vi "FipsAdjacent.vi"() -> (11 "Fips":i32[](array[numeric]))   [LabVIEW 2017] (continued)
County, MD\"\t24043\t\"Washington County, MD\"\t24043\n\"Washington County, MD\"\t24043\t\"Franklin County, PA\"\t42055\n\"Washington County, MD\"\t24043\t\"Fulton County, PA\"\t42057\n\"Washington County, MD\"\t24043\t\"Loudoun County, VA\"\t51107\n\"Washington County, MD\"\t24043\t\"Berkeley County, WV\"\t54003\n\"Washington County, MD\"\t24043\t\"Jefferson County, WV\"\t54037\n\"Washington County, MD\"\t24043\t\"Morgan County, WV\"\t54065\n\"Wicomico County, MD\"\t24045\t\"Sussex County, DE\"\t10005\n\"Wicomico County, MD\"\t24045\t\"Dorchester County, MD\"\t24019\n\"Wicomico County, MD\"\t24045\t\"Somerset County, MD\"\t24039\n\"Wicomico County, MD\"\t24045\t\"Wicomico County, MD\"\t24045\n\"Wicomico County, MD\"\t24045\t\"Worcester County, MD\"\t24047\n\"Worcester County, MD\"\t24047\t\"Sussex County, DE\"\t10005\n\"Worcester County, MD\"\t24047\t\"Somerset County, MD\"\t24039\n\"Worcester County, MD\"\t24047\t\"Wicomico County, MD\"\t24045\n\"Worcester County, MD\"\t24047\t\"Worcester County, MD\"\t24047\n\"Worcester County, MD\"\t24047\t\"Accomack County, VA\"\t51001\n\"Baltimore city, MD\"\t24510\t\"Anne Arundel County, MD\"\t24003\n\"Baltimore city, MD\"\t24510\t\"Baltimore County, MD\"\t24005\n\"Baltimore city, MD\"\t24510\t\"Baltimore city, MD\"\t24510\n\"Barnstable County, MA\"\t25001\t\"Barnstable County, MA\"\t25001\n\"Barnstable County, MA\"\t25001\t\"Bristol County, MA\"\t25005\n\"Barnstable County, MA\"\t25001\t\"Dukes County, MA\"\t25007\n\"Barnstable County, MA\"\t25001\t\"Plymouth County, MA\"\t25023\n\"Berkshire County, MA\"\t25003\t\"Litchfield County, CT\"\t09005\n\"Berkshire County, MA\"\t25003\t\"Berkshire County, MA\"\t25003\n\"Berkshire County, MA\"\t25003\t\"Franklin County, MA\"\t25011\n\"Berkshire County, MA\"\t25003\t\"Hampden County, MA\"\t25013\n\"Berkshire County, MA\"\t25003\t\"Hampshire County, MA\"\t25015\n\"Berkshire County, MA\"\t25003\t\"Columbia County, NY\"\t36021\n\"Berkshire County, MA\"\t25003\t\"Dutchess County, NY\"\t36027\n\"Berkshire County, MA\"\t25003\t\"Rensselaer County, NY\"\t36083\n\"Berkshire County, MA\"\t25003\t\"Bennington County, VT\"\t50003\n\"Bristol County, MA\"\t25005\t\"Barnstable County, MA\"\t25001\n\"Bristol County, MA\"\t25005\t\"Bristol County, MA\"\t25005\n\"Bristol County, MA\"\t25005\t\"Dukes County, MA\"\t25007\n\"Bristol County, MA\"\t25005\t\"Norfolk County, MA\"\t25021\n\"Bristol County, MA\"\t25005\t\"Plymouth County, MA\"\t25023\n\"Bristol County, MA\"\t25005\t\"Bristol County, RI\"\t44001\n\"Bristol County, MA\"\t25005\t\"Newport County, RI\"\t44005\n\"Bristol County, MA\"\t25005\t\"Providence County, RI\"\t44007\n\"Dukes County, MA\"\t25007\t\"Barnstable County, MA\"\t25001\n\"Dukes County, MA\"\t25007\t\"Bristol County, MA\"\t25005\n\"Dukes County, MA\"\t25007\t\"Dukes County, MA\"\t25007\n\"Dukes County, MA\"\t25007\t\"Nantucket County, MA\"\t25019\n\"Essex County, MA\"\t25009\t\"Essex County, MA\"\t25009\n\"Essex County, MA\"\t25009\t\"Middlesex County, MA\"\t25017\n\"Essex County, MA\"\t25009\t\"Suffolk County, MA\"\t25025\n\"Essex County, MA\"\t25009\t\"Hillsborough County, NH\"\t33011\n\"Essex County, MA\"\t25009\t\"Rockingham County, NH\"\t33015\n\"Franklin County, MA\"\t25011\t\"Berkshire County, MA\"\t25003\n\"Franklin County, MA\"\t25011\t\"Franklin County, MA\"\t25011\n\"Franklin County, MA\"\t25011\t\"Hampshire County, MA\"\t25015\n\"Franklin County, MA\"\t25011\t\"Worcester County, MA\"\t25027\n\"Franklin County, MA\"\t25011\t\"Cheshire County, NH\"\t33005\n\"Franklin County, MA\"\t25011\t\"Bennington County, VT\"\t50003\n\"Franklin County, MA\"\t25011\t\"Windham County, VT\"\t50025\n\"Hampden County, MA\"\t25013\t\"Hartford County, CT\"\t09003\n\"Hampden County, MA\"\t25013\t\"Litchfield County, CT\"\t09005\n\"Hampden County, MA\"\t25013\t\"Tolland County, CT\"\t09013\n\"Hampden County, MA\"\t25013\t\"Berkshire County, MA\"\t25003\n\"Hampden County, MA\"\t25013\t\"Hampden County, MA\"\t25013\n\"Hampden County, MA\"\t25013\t\"Hampshire County, MA\"\t25015\n\"Hampden County, MA\"\t25013\t\"Worcester County, MA\"\t25027\n\"Hampshire County, MA\"\t25015\t\"Berkshire County, MA\"\t25003\n\"Hampshire County, MA\"\t25015\t\"Franklin County, MA\"\t25011\n\"Hampshire County, MA\"\t25015\t\"Hampden County, MA\"\t25013\n\"Hampshire County, MA\"\t25015\t\"Hampshire County, MA\"\t25015\n\"Hampshire County, MA\"\t25015\t\"Worcester County, MA\"\t25027\n\"Middlesex County, MA\"\t25017\t\"Essex County, MA\"\t25009\n\"Middlesex County, MA\"\t25017\t\"Middlesex County, MA\"\t25017\n\"Middlesex County, MA\"\t25017\t\"Norfolk County, MA\"\t25021\n\"Middlesex County, MA\"\t25017\t\"Suffolk County, MA\"\t25025\n\"Middlesex County, MA\"\t25017\t\"Worcester County, MA\"\t25027\n\"Middlesex County, MA\"\t25017\t\"Hillsborough County, NH\"\t33011\n\"Nantucket County, MA\"\t25019\t\"Dukes County, MA\"\t25007\n\"Nantucket County, MA\"\t25019\t\"Nantucket County, MA\"\t25019\n\"Norfolk County, MA\"\t25021\t\"Bristol County, MA\"\t25005\n\"Norfolk County, MA\"\t25021\t\"Middlesex County, MA\"\t25017\n\"Norfolk County, MA\"\t25021\t\"Norfolk County, MA\"\t25021\n\"Norfolk County, MA\"\t25021\t\"Plymouth County, MA\"\t25023\n\"Norfolk County, MA\"\t25021\t\"Suffolk County, MA\"\t25025\n\"Norfolk County, MA\"\t25021\t\"Worcester County, MA\"\t25027\n\"Norfolk County, MA\"\t25021\t\"Providence County, RI\"\t44007\n\"Plymouth County, MA\"\t25023\t\"Barnstable County, MA\"\t25001\n\"Plymouth County, MA\"\t25023\t\"Bristol County, MA\"\t25005\n\"Plymouth County, MA\"\t25023\t\"Norfolk County, MA\"\t25021\n\"Plymouth County, MA\"\t25023\t\"Plymouth County, MA\"\t25023\n\"Plymouth County, MA\"\t25023\t\"Suffolk County, MA\"\t25025\n\"Suffolk County, MA\"\t25025\t\"Essex County, MA\"\t25009\n\"Suffolk County, MA\"\t25025\t\"Middlesex County, MA\"\t25017\n\"Suffolk County, MA\"\t25025\t\"Norfolk County, MA\"\t25021\n\"Suffolk County, MA\"\t25025\t\"Plymouth County, MA\"\t25023\n\"Suffolk County, MA\"\t25025\t\"Suffolk County, MA\"\t25025\n\"Worcester County, MA\"\t25027\t\"Tolland County, CT\"\t09013\n\"Worcester County, MA\"\t25027\t\"Windham County, CT\"\t09015\n\"Worcester County, MA\"\t25027\t\"Franklin County, MA\"\t25011\n\"Worcester County, MA\"\t25027\t\"Hampden County, MA\"\t25013\n\"Worcester County, MA\"\t25027\t\"Hampshire County, MA\"\t25015\n\"Worcester County, MA\"\t25027\t\"Middlesex County, MA\"\t25017\n\"Worcester County, MA\"\t25027\t\"Norfolk County, MA\"\t25021\n\"Worcester County, MA\"\t25027\t\"Worcester County, MA\"\t25027\n\"Worcester County, MA\"\t25027\t\"Cheshire County, NH\"\t33005\n\"Worcester County, MA\"\t25027\t\"Hillsborough County, NH\"\t33011\n\"Worcester County, MA\"\t25027\t\"Providence County, RI\"\t44007\n\"Alcona County, MI\"\t26001\t\"Alcona County, MI\"\t26001\n\"Alcona County, MI\"\t26001\t\"Alpena County, MI\"\t26007\n\"Alcona County, MI\"\t26001\t\"Iosco County, MI\"\t26069\n\"Alcona County, MI\"\t26001\t\"Montmorency County, MI\"\t26119\n\"Alcona County, MI\"\t26001\t\"Ogemaw County, MI\"\t26129\n\"Alcona County, MI\"\t26001\t\"Oscoda County, MI\"\t26135\n\"Alger County, MI\"\t26003\t\"Alger County, MI\"\t26003\n\"Alger County, MI\"\t26003\t\"Delta County, MI\"\t26041\n\"Alger County, MI\"\t26003\t\"Keweenaw County, MI\"\t26083\n\"Alger County, MI\"\t26003\t\"Luce County, MI\"\t26095\n\"Alger County, MI\"\t26003\t\"Marquette County, MI\"\t26103\n\"Alger County, MI\"\t26003\t\"Schoolcraft County, MI\"\t26153\n\"Allegan County, MI\"\t26005\t\"Lake County, IL\"\t17097\n\"Allegan County, MI\"\t26005\t\"Allegan County, MI\"\t26005\n\"Allegan County, MI\"\t26005\t\"Barry County, MI\"\t26015\n\"Allegan County, MI\"\t26005\t\"Kalamazoo County, MI\"\t26077\n\"Allegan County, MI\"\t26005\t\"Kent County, MI\"\t26081\n\"Allegan County, MI\"\t26005\t\"Ottawa County, MI\"\t26139\n\"Allegan County, MI\"\t26005\t\"Van Buren County, MI\"\t26159\n\"Allegan County, MI\"\t26005\t\"Kenosha County, WI\"\t55059\n\"Allegan County, MI\"\t26005\t\"Racine County, WI\"\t55101\n\"Alpena County, MI\"\t26007\t\"Alcona County, MI\"\t26001\n\"Alpena County, MI\"\t26007\t\"Alpena County, MI\"\t26007\n\"Alpena County, MI\"\t26007\t\"Montmorency County, MI\"\t26119\n\"Alpena County, MI\"\t26007\t\"Oscoda County, MI\"\t26135\n\"Alpena County, MI\"\t26007\t\"Presque Isle County, MI\"\t26141\n\"Antrim County, MI\"\t26009\t\"Antrim County, MI\"\t26009\n\"Antrim County, MI\"\t26009\t\"Charlevoix County, MI\"\t26029\n\"Antrim County, MI\"\t26009\t\"Crawford County, MI\"\t26039\n\"Antrim County, MI\"\t26009\t\"Grand Traverse County, MI\"\t26055\n\"Antrim County, MI\"\t26009\t\"Kalkaska County, MI\"\t26079\n\"Antrim County, MI\"\t26009\t\"Leelanau County, MI\"\t26089\n\"Antrim County, MI\"\t26009\t\"Otsego County, MI\"\t26137\n\"Arenac County, MI\"\t26011\t\"Arenac County, MI\"\t26011\n\"Arenac County, MI\"\t26011\t\"Bay County, MI\"\t26017\n\"Arenac County, MI\"\t26011\t\"Gladwin County, MI\"\t26051\n\"Arenac County, MI\"\t26011\t\"Huron County, MI\"\t26063\n\"Arenac County, MI\"\t26011\t\"Iosco County, MI\"\t26069\n\"Arenac County, MI\"\t26011\t\"Ogemaw County, MI\"\t26129\n\"Baraga County, MI\"\t26013\t\"Baraga County, MI\"\t26013\n\"Baraga County, MI\"\t26013\t\"Houghton County, MI\"\t26061\n\"Baraga County, MI\"\t26013\t\"Iron County, MI\"\t26071\n\"Baraga County, MI\"\t26013\t\"Marquette County, MI\"\t26103\n\"Barry County, MI\"\t26015\t\"Allegan County, MI\"\t26005\n\"Barry County, MI\"\t26015\t\"Barry County, MI\"\t26015\n\"Barry County, MI\"\t26015\t\"Calhoun County, MI\"\t26025\n\"Barry County, MI\"\t26015\t\"Eaton County, MI\"\t26045\n\"Barry County, MI\"\t26015\t\"Ionia County, MI\"\t26067\n\"Barry County, MI\"\t26015\t\"Kalamazoo County, MI\"\t26077\n\"Barry County, MI\"\t26015\t\"Kent County, MI\"\t26081\n\"Bay County, MI\"\t26017\t\"Arenac County, MI\"\t26011\n\"Bay County, MI\"\t26017\t\"Bay County, MI\"\t26017\n\"Bay County, MI\"\t26017\t\"Gladwin County, MI\"\t26051\n\"Bay County, MI\"\t26017\t\"Huron County, MI\"\t26063\n\"Bay County, MI\"\t26017\t\"Midland County, MI\"\t26111\n\"Bay County, MI\"\t26017\t\"Saginaw County, MI\"\t26145\n\"Bay County, MI\"\t26017\t\"Tuscola County, MI\"\t26157\n\"Benzie County, MI\"\t26019\t\"Benzie County, MI\"\t26019\n\"Benzie County, MI\"\t26019\t\"Grand Traverse County, MI\"\t26055\n\"Benzie County, MI\"\t26019\t\"Leelanau County, MI\"\t26089\n\"Benzie County, MI\"\t26019\t\"Manistee County, MI\"\t26101\n\"Benzie County, MI\"\t26019\t\"Wexford County, MI\"\t26165\n\"Benzie County, MI\"\t26019\t\"Door County, WI\"\t55029\n\"Benzie County, MI\"\t26019\t\"Kewaunee County, WI\"\t55061\n\"Berrien County, MI\"\t26021\t\"Cook County, IL\"\t17031\n\"Berrien County, MI\"\t26021\t\"Lake County, IL\"\t17097\n\"Berrien County, MI\"\t26021\t\"LaPorte County, IN\"\t18091\n\"Berrien County, MI\"\t26021\t\"Porter County, IN\"\t18127\n\"Berrien County, MI\"\t26021\t\"St. Joseph County, IN\"\t18141\n\"Berrien County, MI\"\t26021\t\"Berrien County, MI\"\t26021\n\"Berrien County, MI\"\t26021\t\"Cass County, MI\"\t26027\n\"Berrien County, MI\"\t26021\t\"Van Buren County, MI\"\t26159\n\"Branch County, MI\"\t26023\t\"LaGrange County, IN\"\t18087\n\"Branch County, MI\"\t26023\t\"Steuben County, IN\"\t18151\n\"Branch County, MI\"\t26023\t\"Branch County, MI\"\t26023\n\"Branch County, MI\"\t26023\t\"Calhoun County, MI\"\t26025\n\"Branch County, MI\"\t26023\t\"Hillsdale County, MI\"\t26059\n\"Branch County, MI\"\t26023\t\"Kalamazoo County, MI\"\t26077\n\"Branch County, MI\"\t26023\t\"St. Joseph County, MI\"\t26149\n\"Calhoun County, MI\"\t26025\t\"Barry County, MI\"\t26015\n\"Calhoun County, MI\"\t26025\t\"Branch County, MI\"\t26023\n\"Calhoun County, MI\"\t26025\t\"Calhoun County, MI\"\t26025\n\"Calhoun County, MI\"\t26025\t\"Eaton County, MI\"\t26045\n\"Calhoun County, MI\"\t26025\t\"Hillsdale County, MI\"\t26059\n\"Calhoun County, MI\"\t26025\t\"Jackson County, MI\"\t26075\n\"Calhoun County, MI\"\t26025\t\"Kalamazoo County, MI\"\t26077\n\"Calhoun County, MI\"\t26025\t\"St. Joseph County, MI\"\t26149\n\"Cass County, MI\"\t26027\t\"Elkhart County, IN\"\t18039\n\"Cass County, MI\"\t26027\t\"St. Joseph County, IN\"\t18141\n\"Cass County, MI\"\t26027\t\"Berrien County, MI\"\t26021\n\"Cass County, MI\"\t26027\t\"Cass County, MI\"\t26027\n\"Cass County, MI\"\t26027\t\"Kalamazoo County, MI\"\t26077\n\"Cass County, MI\"\t26027\t\"St. Joseph County, MI\"\t26149\n\"Cass County, MI\"\t26027\t\"Van Buren County, MI\"\t26159\n\"Charlevoix County, MI\"\t26029\t\"Antrim County, MI\"\t26009\n\"Charlevoix County, MI\"\t26029\t\"Charlevoix County, MI\"\t26029\n\"Charlevoix County, MI\"\t26029\t\"Cheboygan County, MI\"\t26031\n\"Charlevoix County, MI\"\t26029\t\"Emmet County, MI\"\t26047\n\"Charlevoix County, MI\"\t26029\t\"Leelanau County, MI\"\t26089\n\"Charlevoix County, MI\"\t26029\t\"Mackinac County, MI\"\t26097\n\"Charlevoix County, MI\"\t26029\t\"Otsego County, MI\"\t26137\n\"Charlevoix County, MI\"\t26029\t\"Schoolcraft County, MI\"\t26153\n\"Cheboygan County, MI\"\t26031\t\"Charlevoix County, MI\"\t26029\n\"Cheboygan County, MI\"\t26031\t\"Cheboygan County, MI\"\t26031\n\"Cheboygan County, MI\"\t26031\t\"Emmet County, MI\"\t26047\n\"Cheboygan County, MI\"\t26031\t\"Mackinac County, MI\"\t26097\n\"Cheboygan County, MI\"\t26031\t\"Montmorency County, MI\"\t26119\n\"Cheboygan County, MI\"\t26031\t\"Otsego County, MI\"\t26137\n\"Cheboygan County, MI\"\t26031\t\"Presque Isle County, MI\"\t26141\n\"Chippewa County, MI\"\t26033\t\"Chippewa County, MI\"\t26033\n\"Chippewa County, MI\"\t26033\t\"Luce County, MI\"\t26095\n\"Chippewa County, MI\"\t26033\t\"Mackinac County, MI\"\t26097\n\"Chippewa County, MI\"\t26033\t\"Presque Isle County, MI\"\t26141\n\"Clare County, MI\"\t26035\t\"Clare County, MI\"\t26035\n\"Clare County, MI\"\t26035\t\"Gladwin County, MI\"\t26051\n\"Clare County, MI\"\t26035\t\"Isabella County, MI\"\t26073\n\"Clare County, MI\"\t26035\t\"Mecosta County, MI\"\t26107\n\"Clare County, MI\"\t26035\t\"Midland County, MI\"\t26111\n\"Clare County, MI\"\t26035\t\"Missaukee County, MI\"\t26113\n\"Clare County, MI\"\t26035\t\"Osceola County, MI\"\t26133\n\"Clare County, MI\"\t26035\t\"Roscommon County, MI\"\t26143\n\"Clinton County, MI\"\t26037\t\"Clinton County, MI\"\t26037\n\"Clinton County, MI\"\t26037\t\"Eaton County, MI\"\t26045\n\"Clinton County, MI\"\t26037\t\"Gratiot County, MI\"\t26057\n\"Clinton County, MI\"\t26037\t\"Ingham County, MI\"\t26065\n\"Clinton County, MI\"\t26037\t\"Ionia County, MI\"\t26067\n\"Clinton County, MI\"\t26037\t\"Montcalm County, MI\"\t26117\n\"Clinton County, MI\"\t26037\t\"Shiawassee County, MI\"\t26155\n\"Crawford County, MI\"\t26039\t\"Antrim County, MI\"\t26009\n\"Crawford County, MI\"\t26039\t\"Crawford County, MI\"\t26039\n\"Crawford County, MI\"\t26039\t\"Kalkaska County, MI\"\t26079\n\"Crawford County, MI\"\t26039\t\"Missaukee County, MI\"\t26113\n\"Crawford County, MI\"\t26039\t\"Montmorency County, MI\"\t26119\n\"Crawford County, MI\"\t26039\t\"Ogemaw County, MI\"\t26129\n\"Crawford County, MI\"\t26039\t\"Oscoda County, MI\"\t26135\n\"Crawford County, MI\"\t26039\t\"Otsego County, MI\"\t26137\n\"Crawford County, MI\"\t26039\t\"Roscommon County, MI\"\t26143\n\"Delta County, MI\"\t26041\t\"Alger County, MI\"\t26003\n\"Delta County, MI\"\t26041\t\"Delta County, MI\"\t26041\n\"Delta County, MI\"\t26041\t\"Leelanau County, MI\"\t26089\n\"Delta County, MI\"\t26041\t\"Marquette County, MI\"\t26103\n\"Delta County, MI\"\t26041\t\"Menominee County, MI\"\t26109\n\"Delta County, MI\"\t26041\t\"Schoolcraft County, MI\"\t26153\n\"Delta County, MI\"\t26041\t\"Door County, WI\"\t55029\n\"Dickinson County, MI\"\t26043\t\"Dickinson County, MI\"\t26043\n\"Dickinson County, MI\"\t26043\t\"Iron County, MI\"\t26071\n\"Dickinson County, MI\"\t26043\t\"Marquette County, MI\"\t26103\n\"Dickinson County, MI\"\t26043\t\"Menominee County, MI\"\t26109\n\"Dickinson County, MI\"\t26043\t\"Florence County, WI\"\t55037\n\"Dickinson County, MI\"\t26043\t\"Marinette County, WI\"\t55075\n\"Eaton County, MI\"\t26045\t\"Barry County, MI\"\t26015\n\"Eaton County, MI\"\t26045\t\"Calhoun County, MI\"\t26025\n\"Eaton County, MI\"\t26045\t\"Clinton County, MI\"\t26037\n\"Eaton County, MI\"\t26045\t\"Eaton County, MI\"\t26045\n\"Eaton County, MI\"\t26045\t\"Ingham County, MI\"\t26065\n\"Eaton County, MI\"\t26045\t\"Ionia County, MI\"\t26067\n\"Eaton County, MI\"\t26045\t\"Jackson County, MI\"\t26075\n\"Emmet County, MI\"\t26047\t\"Charlevoix County, MI\"\t26029\n\"Emmet County, MI\"\t26047\t\"Cheboygan County, MI\"\t26031\n\"Emmet County, MI\"\t26047\t\"Emmet County, MI\"\t26047\n\"Emmet County, MI\"\t26047\t\"Mackinac County, MI\"\t26097\n\"Genesee County, MI\"\t26049\t\"Genesee County, MI\"\t26049\n\"Genesee County, MI\"\t26049\t\"Lapeer County, MI\"\t26087\n\"Genesee County, MI\"\t26049\t\"Livingston County, MI\"\t26093\n\"Genesee County, MI\"\t26049\t\"Oakland County, MI\"\t26125\n\"Genesee County, MI\"\t26049\t\"Saginaw County, MI\"\t26145\n\"Genesee County, MI\"\t26049\t\"Shiawassee County, MI\"\t26155\n\"Genesee County, MI\"\t26049\t\"Tuscola County, MI\"\t26157\n\"Gladwin County, MI\"\t26051\t\"Arenac County, MI\"\t26011\n\"Gladwin County, MI\"\t26051\t\"Bay County, MI\"\t26017\n\"Gladwin County, MI\"\t26051\t\"Clare County, MI\"\t26035\n\"Gladwin County, MI\"\t26051\t\"Gladwin County, MI\"\t26051\n\"Gladwin County, MI\"\t26051\t\"Isabella County, MI\"\t26073\n\"Gladwin County, MI\"\t26051\t\"Midland County, MI\"\t26111\n\"Gladwin County, MI\"\t26051\t\"Ogemaw County, MI\"\t26129\n\"Gladwin County, MI\"\t26051\t\"Roscommon County, MI\"\t26143\n\"Gogebic County, MI\"\t26053\t\"Gogebic County, MI\"\t26053\n\"Gogebic County, MI\"\t26053\t\"Iron County, MI\"\t26071\n\"Gogebic County, MI\"\t26053\t\"Ontonagon County, MI\"\t26131\n\"Gogebic County, MI\"\t26053\t\"Ashland County, WI\"\t55003\n\"Gogebic County, MI\"\t26053\t\"Iron County, WI\"\t55051\n\"Gogebic County, MI\"\t26053\t\"Vilas County, WI\"\t55125\n\"Grand Traverse County, MI\"\t26055\t\"Antrim County, MI\"\t26009\n\"Grand Traverse County, MI\"\t26055\t\"Benzie County, MI\"\t26019\n\"Grand Traverse County, MI\"\t26055\t\"Grand Traverse County, MI\"\t26055\n\"Grand Traverse County, MI\"\t26055\t\"Kalkaska County, MI\"\t26079\n\"Grand Traverse County, MI\"\t26055\t\"Leelanau County, MI\"\t26089\n\"Grand Traverse County, MI\"\t26055\t\"Manistee County, MI\"\t26101\n\"Grand Traverse County, MI\"\t26055\t\"Missaukee County, MI\"\t26113\n\"Grand Traverse County, MI\"\t26055\t\"Wexford County, MI\"\t26165\n\"Gratiot County, MI\"\t26057\t\"Clinton County, MI\"\t26037\n\"Gratiot County, MI\"\t26057\t\"Gratiot County, MI\"\t26057\n\"Gratiot County, MI\"\t26057\t\"Ionia County, MI\"\t26067\n\"Gratiot County, MI\"\t26057\t\"Isabella County, MI\"\t26073\n\"Gratiot County, MI\"\t26057\t\"Midland County, MI\"\t26111\n\"Gratiot County, MI\"\t26057\t\"Montcalm County, MI\"\t26117\n\"Gratiot County, MI\"\t26057\t\"Saginaw County, MI\"\t26145\n\"Gratiot County, MI\"\t26057\t\"Shiawassee County, MI\"\t26155\n\"Hillsdale County, MI\"\t26059\t\"Steuben County, IN\"\t18151\n\"Hillsdale County, MI\"\t26059\t\"Branch County, MI\"\t26023\n\"Hillsdale County, MI\"\t26059\t\"Calhoun County, MI\"\t26025\n\"Hillsdale County, MI\"\t26059\t\"Hillsdale County, MI\"\t26059\n\"Hillsdale County, MI\"\t26059\t\"Jackson County, MI\"\t26075\n\"Hillsdale County, MI\"\t26059\t\"Lenawee County, MI\"\t26091\n\"Hillsdale County, MI\"\t26059\t\"Fulton County, OH\"\t39051\n\"Hillsdale County, MI\"\t26059\t\"Williams County, OH\"\t39171\n\"Houghton County, MI\"\t26061\t\"Baraga County, MI\"\t26013\n\"Houghton County, MI\"\t26061\t\"Houghton County, MI\"\t26061\n\"Houghton County, MI\"\t26061\t\"Iron County, MI\"\t26071\n\"Houghton County, MI\"\t26061\t\"Keweenaw County, MI\"\t26083\n\"Houghton County, MI\"\t26061\t\"Marquette County, MI\"\t26103\n\"Houghton County, MI\"\t26061\t\"Ontonagon County, MI\"\t26131\n\"Huron County, MI\"\t26063\t\"Arenac County, MI\"\t26011\n\"Huron County, MI\"\t26063\t\"Bay County, MI\"\t26017\n\"Huron County, MI\"\t26063\t\"Huron County, MI\"\t26063\n\"Huron County, MI\"\t26063\t\"Iosco County, MI\"\t26069\n\"Huron County, MI\"\t26063\t\"Sanilac County, MI\"\t26151\n\"Huron County, MI\"\t26063\t\"Tuscola County, MI\"\t26157\n\"Ingham County, MI\"\t26065\t\"Clinton County, MI\"\t26037\n\"Ingham County, MI\"\t26065\t\"Eaton County, MI\"\t26045\n\"Ingham County, MI\"\t26065\t\"Ingham County, MI\"\t26065\n\"Ingham County, MI\"\t26065\t\"Jackson County, MI\"\t26075\n\"Ingham County, MI\"\t26065\t\"Livingston County, MI\"\t26093\n\"Ingham County, MI\"\t26065\t\"Shiawassee County, MI\"\t26155\n\"Ionia County, MI\"\t26067\t\"Barry County, MI\"\t26015\n\"Ionia County, MI\"\t26067\t\"Clinton County, MI\"\t26037\n\"Ionia County, MI\"\t26067\t\"Eaton County, MI\"\t26045\n\"Ionia County, MI\"\t26067\t\"Gratiot County, MI\"\t26057\n\"Ionia County, MI\"\t26067\t\"Ionia County, MI\"\t26067\n\"Ionia County, MI\"\t26067\t\"Kent County, MI\"\t26081\n\"Ionia County, MI\"\t26067\t\"Montcalm County, MI\"\t26117\n\"Iosco County, MI\"\t26069\t\"Alcona County, MI\"\t26001\n\"Iosco County, MI\"\t26069\t\"Arenac County, MI\"\t26011\n\"Iosco County, MI\"\t26069\t\"Huron County, MI\"\t26063\n\"Iosco County, MI\"\t26069\t\"Iosco County, MI\"\t26069\n\"Iosco County, MI\"\t26069\t\"Ogemaw County, MI\"\t26129\n\"Iosco County, MI\"\t26069\t\"Oscoda County, MI\"\t26135\n\"Iron County, MI\"\t26071\t\"Baraga County, MI\"\t26013\n\"Iron County, MI\"\t26071\t\"Dickinson County, MI\"\t26043\n\"Iron County, MI\"\t26071\t\"Gogebic County, MI\"\t26053\n\"Iron County, MI\"\t26071\t\"Houghton County, MI\"\t26061\n\"Iron County, MI\"\t26071\t\"Iron County, MI\"\t26071\n\"Iron County, MI\"\t26071\t\"Marquette County, MI\"\t26103\n\"Iron County, MI\"\t26071\t\"Ontonagon County, MI\"\t26131\n\"Iron County, MI\"\t26071\t\"Florence County, WI\"\t55037\n\"Iron County, MI\"\t26071\t\"Forest County, WI\"\t55041\n\"Iron County, MI\"\t26071\t\"Vilas County, WI\"\t55125\n\"Isabella County, MI\"\t26073\t\"Clare County, MI\"\t26035\n\"Isabella County, MI\"\t26073\t\"Gladwin County, MI\"\t26051\n\"Isabella County, MI\"\t26073\t\"Gratiot County, MI\"\t26057\n\"Isabella County, MI\"\t26073\t\"Isabella County, MI\"\t26073\n\"Isabella County, MI\"\t26073\t\"Mecosta County, MI\"\t26107\n\"Isabella County, MI\"\t26073\t\"Midland County, MI\"\t26111\n\"Isabella County, MI\"\t26073\t\"Montcalm County, MI\"\t26117\n\"Isabella County, MI\"\t26073\t\"Osceola County, MI\"\t26133\n\"Jackson County, MI\"\t26075\t\"Calhoun County, MI\"\t26025\n\"Jackson County, MI\"\t26075\t\"Eaton County, MI\"\t26045\n\"Jackson County, MI\"\t26075\t\"Hillsdale County, MI\"\t26059\n\"Jackson County, MI\"\t26075\t\"Ingham County, MI\"\t26065\n\"Jackson County, MI\"\t26075\t\"Jackson County, MI\"\t26075\n\"Jackson County, MI\"\t26075\t\"Lenawee County, MI\"\t26091\n\"Jackson County, MI\"\t26075\t\"Livingston County, MI\"\t26093\n\"Jackson County, MI\"\t26075\t\"Washtenaw County, MI\"\t26161\n\"Kalamazoo County, MI\"\t26077\t\"Allegan County, MI\"\t26005\n\"Kalamazoo County, MI\"\t26077\t\"Barry County, MI\"\t26015\n\"Kalamazoo County, MI\"\t26077\t\"Branch County, MI\"\t26023\n\"Kalamazoo County, MI\"\t26077\t\"Calhoun County, MI\"\t26025\n\"Kalamazoo County, MI\"\t26077\t\"Cass County, MI\"\t26027\n\"Kalamazoo County, MI\"\t26077\t\"Kalamazoo County, MI\"\t26077\n\"Kalamazoo County, MI\"\t26077\t\"St. Joseph County, MI\"\t26149\n\"Kalamazoo County, MI\"\t26077\t\"Van Buren County, MI\"\t26159\n\"Kalkaska County, MI\"\t26079\t\"Antrim County, MI\"\t26009\n\"Kalkaska County, MI\"\t26079\t\"Crawford County, MI\"\t26039\n\"Kalkaska County, MI\"\t26079\t\"Grand Traverse County, MI\"\t26055\n\"Kalkaska County, MI\"\t26079\t\"Kalkaska County, MI\"\t26079\n\"Kalkaska County, MI\"\t26079\t\"Missaukee County, MI\"\t26113\n\"Kalkaska County, MI\"\t26079\t\"Otsego County, MI\"\t26137\n\"Kalkaska County, MI\"\t26079\t\"Roscommon County, MI\"\t26143\n\"Kalkaska County, MI\"\t26079\t\"Wexford County, MI\"\t26165\n\"Kent County, MI\"\t26081\t\"Allegan County, MI\"\t26005\n\"Kent County, MI\"\t26081\t\"Barry County, MI\"\t26015\n\"Kent County, MI\"\t26081\t\"Ionia County, MI\"\t26067\n\"Kent County, MI\"\t26081\t\"Kent County, MI\"\t26081\n\"Kent County, MI\"\t26081\t\"Montcalm County, MI\"\t26117\n\"Kent County, MI\"\t26081\t\"Muskegon County, MI\"\t26121\n\"Kent County, MI\"\t26081\t\"Newaygo County, MI\"\t26123\n\"Kent County, MI\"\t26081\t\"Ottawa County, MI\"\t26139\n\"Keweenaw County, MI\"\t26083\t\"Alger County, MI\"\t26003\n\"Keweenaw County, MI\"\t26083\t\"Houghton County, MI\"\t26061\n\"Keweenaw County, MI\"\t26083\t\"Keweenaw County, MI\"\t26083\n\"Keweenaw County, MI\"\t26083\t\"Marquette County, MI\"\t26103\n\"Keweenaw County, MI\"\t26083\t\"Ontonagon County, MI\"\t26131\n\"Keweenaw County, MI\"\t26083\t\"Cook County, MN\"\t27031\n\"Lake County, MI\"\t26085\t\"Lake County, MI\"\t26085\n\"Lake County, MI\"\t26085\t\"Manistee County, MI\"\t26101\n\"Lake County, MI\"\t26085\t\"Mason County, MI\"\t26105\n\"Lake County, MI\"\t26085\t\"Mecosta County, MI\"\t26107\n\"Lake County, MI\"\t26085\t\"Newaygo County, MI\"\t26123\n\"Lake County, MI\"\t26085\t\"Oceana County, MI\"\t26127\n\"Lake County, MI\"\t26085\t\"Osceola County, MI\"\t26133\n\"Lake County, MI\"\t26085\t\"Wexford County, MI\"\t26165\n\"Lapeer County, MI\"\t26087\t\"Genesee County, MI\"\t26049\n\"Lapeer County, MI\"\t26087\t\"Lapeer County, MI\"\t26087\n\"Lapeer County, MI\"\t26087\t\"Macomb County, MI\"\t26099\n\"Lapeer County, MI\"\t26087\t\"Oakland County, MI\"\t26125\n\"Lapeer County, MI\"\t26087\t\"St. Clair County, MI\"\t26147\n\"Lapeer County, MI\"\t26087\t\"Sanilac County, MI\"\t26151\n\"Lapeer County, MI\"\t26087\t\"Tuscola County, MI\"\t26157\n\"Leelanau County, MI\"\t26089\t\"Antrim County, MI\"\t26009\n\"Leelanau County, MI\"\t26089\t\"Benzie County, MI\"\t26019\n\"Leelanau County, MI\"\t26089\t\"Charlevoix County, MI\"\t26029\n\"Leelanau County, MI\"\t26089\t\"Delta County, MI\"\t26041\n\"Leelanau County, MI\"\t26089\t\"Grand Traverse County, MI\"\t26055\n\"Leelanau County, MI\"\t26089\t\"Leelanau County, MI\"\t26089\n\"Leelanau County, MI\"\t26089\t\"Schoolcraft County, MI\"\t26153\n\"Leelanau County, MI\"\t26089\t\"Door County, WI\"\t55029\n\"Lenawee County, MI\"\t26091\t\"Hillsdale County, MI\"\t26059\n\"Lenawee County, MI\"\t26091\t\"Jackson County, MI\"\t26075\n\"Lenawee County, MI\"\t26091\t\"Lenawee County, MI\"\t26091\n\"Lenawee County, MI\"\t26091\t\"Monroe County, MI\"\t26115\n\"Lenawee County, MI\"\t26091\t\"Washtenaw County, MI\"\t26161\n\"Lenawee County, MI\"\t26091\t\"Fulton County, OH\"\t39051\n\"Lenawee County, MI\"\t26091\t\"Lucas County, OH\"\t39095\n\"Livingston County, MI\"\t26093\t\"Genesee County, MI\"\t26049\n\"Livingston County, MI\"\t26093\t\"Ingham County, MI\"\t26065\n\"Livingston County, MI\"\t26093\t\"Jackson County, MI\"\t26075\n\"Livingston County, MI\"\t26093\t\"Livingston County, MI\"\t26093\n\"Livingston County, MI\"\t26093\t\"Oakland County, MI\"\t26125\n\"Livingston County, MI\"\t26093\t\"Shiawassee County, MI\"\t26155\n\"Livingston County, MI\"\t26093\t\"Washtenaw County, MI\"\t26161\n\"Luce County, MI\"\t26095\t\"Alger County, MI\"\t26003\n\"Luce County, MI\"\t26095\t\"Chippewa County, MI\"\t26033\n\"Luce County, MI\"\t26095\t\"Luce County, MI\"\t26095\n\"Luce County, MI\"\t26095\t\"Mackinac County, MI\"\t26097\n\"Luce County, MI\"\t26095\t\"Schoolcraft County, MI\"\t26153\n\"Mackinac County, MI\"\t26097\t\"Charlevoix County, MI\"\t26029\n\"Mackinac County, MI\"\t26097\t\"Cheboygan County, MI\"\t26031\n\"Mackinac County, MI\"\t26097\t\"Chippewa County, MI\"\t26033\n\"Mackinac County, MI\"\t26097\t\"Emmet County, MI\"\t26047\n\"Mackinac County, MI\"\t26097\t\"Luce County, MI\"\t26095\n\"Mackinac County, MI\"\t26097\t\"Mackinac County, MI\"\t26097\n\"Mackinac County, MI\"\t26097\t\"Presque Isle County, MI\"\t26141\n\"Mackinac County, MI\"\t26097\t\"Schoolcraft County, MI\"\t26153\n\"Macomb County, MI\"\t26099\t\"Lapeer County, MI\"\t26087\n\"Macomb County, MI\"\t26099\t\"Macomb County, MI\"\t26099\n\"Macomb County, MI\"\t26099\t\"Oakland County, MI\"\t26125\n\"Macomb County, MI\"\t26099\t\"St. Clair County, MI\"\t26147\n\"Macomb County, MI\"\t26099\t\"Wayne County, MI\"\t26163\n\"Manistee County, MI\"\t26101\t\"Benzie County, MI\"\t26019\n\"Manistee County, MI\"\t26101\t\"Grand Traverse County, MI\"\t26055\n\"Manistee County, MI\"\t26101\t\"Lake County, MI\"\t26085\n\"Manistee County, MI\"\t26101\t\"Manistee County, MI\"\t26101\n\"Manistee County, MI\"\t26101\t\"Mason County, MI\"\t26105\n\"Manistee County, MI\"\t26101\t\"Wexford County, MI\"\t26165\n\"Manistee County, MI\"\t26101\t\"Kewaunee County, WI\"\t55061\n\"Manistee County, MI\"\t26101\t\"Manitowoc County, WI\"\t55071\n\"Marquette County, MI\"\t26103\t\"Alger County, MI\"\t26003\n\"Marquette County, MI\"\t26103\t\"Baraga County, MI\"\t26013\n\"Marquette County, MI\"\t26103\t\"Delta County, MI\"\t26041\n\"Marquette County, MI\"\t26103\t\"Dickinson County, MI\"\t26043\n\"Marquette County, MI\"\t26103\t\"Houghton County, MI\"\t26061\n\"Marquette County, MI\"\t26103\t\"Iron County, MI\"\t26071\n\"Marquette County, MI\"\t26103\t\"Keweenaw County, MI\"\t26083\n\"Marquette County, MI\"\t26103\t\"Marquette County, MI\"\t26103\n\"Marquette County, MI\"\t26103\t\"Menominee County, MI\"\t26109\n\"Mason County, MI\"\t26105\t\"Lake County, MI\"\t26085\n\"Mason County, MI\"\t26105\t\"Manistee County, MI\"\t26101\n\"Mason County, MI\"\t26105\t\"Mason County, MI\"\t26105\n\"Mason County, MI\"\t26105\t\"Newaygo County, MI\"\t26123\n\"Mason County, MI\"\t26105\t\"Oceana County, MI\"\t26127\n\"Mason County, MI\"\t26105\t\"Manitowoc County, WI\"\t55071\n\"Mason County, MI\"\t26105\t\"Sheboygan County, WI\"\t55117\n\"Mecosta County, MI\"\t26107\t\"Clare County, MI\"\t26035\n\"Mecosta County, MI\"\t26107\t\"Isabella County, MI\"\t26073\n\"Mecosta County, MI\"\t26107\t\"Lake County, MI\"\t26085\n\"Mecosta County, MI\"\t26107\t\"Mecosta County, MI\"\t26107\n\"Mecosta County, MI\"\t26107\t\"Montcalm County, MI\"\t26117\n\"Mecosta County, MI\"\t26107\t\"Newaygo County, MI\"\t26123\n\"Mecosta County, MI\"\t26107\t\"Osceola County, MI\"\t26133\n\"Menominee County, MI\"\t26109\t\"Delta County, MI\"\t26041\n\"Menominee County, MI\"\t26109\t\"Dickinson County, MI\"\t26043\n\"Menominee County, MI\"\t26109\t\"Marquette County, MI\"\t26103\n\"Menominee County, MI\"\t26109\t\"Menominee County, MI\"\t26109\n\"Menominee County, MI\"\t26109\t\"Door County, WI\"\t55029\n\"Menominee County, MI\"\t26109\t\"Marinette County, WI\"\t55075\n\"Midland County, MI\"\t26111\t\"Bay County, MI\"\t26017\n\"Midland County, MI\"\t26111\t\"Clare County, MI\"\t26035\n\"Midland County, MI\"\t26111\t\"Gladwin County, MI\"\t26051\n\"Midland County, MI\"\t26111\t\"Gratiot County, MI\"\t26057\n\"Midland County, MI\"\t26111\t\"Isabella County, MI\"\t26073\n\"Midland County, MI\"\t26111\t\"Midland County, MI\"\t26111\n\"Midland County, MI\"\t26111\t\"Saginaw County, MI\"\t26145\n\"Missaukee County, MI\"\t26113\t\"Clare County, MI\"\t26035\n\"Missaukee County, MI\"\t26113\t\"Crawford County, MI\"\t26039\n\"Missaukee County, MI\"\t26113\t\"Grand Traverse County, MI\"\t26055\n\"Missaukee County, MI\"\t26113\t\"Kalkaska County, MI\"\t26079\n\"Missaukee County, MI\"\t26113\t\"Missaukee County, MI\"\t26113\n\"Missaukee County, MI\"\t26113\t\"Osceola County, MI\"\t26133\n\"Missaukee County, MI\"\t26113\t\"Roscommon County, MI\"\t26143\n\"Missaukee County, MI\"\t26113\t\"Wexford County, MI\"\t26165\n\"Monroe County, MI\"\t26115\t\"Lenawee County, MI\"\t26091\n\"Monroe County, MI\"\t26115\t\"Monroe County, MI\"\t26115\n\"Monroe County, MI\"\t26115\t\"Washtenaw County, MI\"\t26161\n\"Monroe County, MI\"\t26115\t\"Wayne County, MI\"\t26163\n\"Monroe County, MI\"\t26115\t\"Lucas County, OH\"\t39095\n\"Montcalm County, MI\"\t26117\t\"Clinton County, MI\"\t26037\n\"Montcalm County, MI\"\t26117\t\"Gratiot County, MI\"\t26057\n\"Montcalm County, MI\"\t26117\t\"Ionia County, MI\"\t26067\n\"Montcalm County, MI\"\t26117\t\"Isabella County, MI\"\t26073\n\"Montcalm County, MI\"\t26117\t\"Kent County, MI\"\t26081\n\"Montcalm County, MI\"\t26117\t\"Mecosta County, MI\"\t26107\n\"Montcalm County, MI\"\t26117\t\"Montcalm County, MI\"\t26117\n\"Montcalm County, MI\"\t26117\t\"Newaygo County, MI\"\t26123\n\"Montmorency County, MI\"\t26119\t\"Alcona County, MI\"\t26001\n\"Montmorency County, MI\"\t26119\t\"Alpena County, MI\"\t26007\n\"Montmorency County, MI\"\t26119\t\"Cheboygan County, MI\"\t26031\n\"Montmorency County, MI\"\t26119\t\"Crawford County, MI\"\t26039\n\"Montmorency County, MI\"\t26119\t\"Montmorency County, MI\"\t26119\n\"Montmorency County, MI\"\t26119\t\"Oscoda County, MI\"\t26135\n\"Montmorency County, MI\"\t26119\t\"Otsego County, MI\"\t26137\n\"Montmorency County, MI\"\t26119\t\"Presque Isle County, MI\"\t26141\n\"Muskegon County, MI\"\t26121\t\"Kent County, MI\"\t26081\n\"Muskegon County, MI\"\t26121\t\"Muskegon County, MI\"\t26121\n\"Muskegon County, MI\"\t26121\t\"Newaygo County, MI\"\t26123\n\"Muskegon County, MI\"\t26121\t\"Oceana County, MI\"\t26127\n\"Muskegon County, MI\"\t26121\t\"Ottawa County, MI\"\t26139\n\"Muskegon County, MI\"\t26121\t\"Milwaukee County, WI\"\t55079\n\"Muskegon County, MI\"\t26121\t\"Ozaukee County, WI\"\t55089\n\"Newaygo County, MI\"\t26123\t\"Kent County, MI\"\t26081\n\"Newaygo County, MI\"\t26123\t\"Lake County, MI\"\t26085\n\"Newaygo County, MI\"\t26123\t\"Mason County, MI\"\t26105\n\"Newaygo County, MI\"\t26123\t\"Mecosta County, MI\"\t26107\n\"Newaygo County, MI\"\t26123\t\"Montcalm County, MI\"\t26117\n\"Newaygo County, MI\"\t26123\t\"Muskegon County, MI\"\t26121\n\"Newaygo County, MI\"\t26123\t\"Newaygo County, MI\"\t26123\n\"Newaygo County, MI\"\t26123\t\"Oceana County, MI\"\t26127\n\"Newaygo County, MI\"\t26123\t\"Osceola County, MI\"\t26133\n\"Oakland County, MI\"\t26125\t\"Genesee County, MI\"\t26049\n\"Oakland County, MI\"\t26125\t\"Lapeer County, MI\"\t26087\n\"Oakland County, MI\"\t26125\t\"Livingston County, MI\"\t26093\n\"Oakland County, MI\"\t26125\t\"Macomb County, MI\"\t26099\n\"Oakland County, MI\"\t26125\t\"Oakland County, MI\"\t26125\n\"Oakland County, MI\"\t26125\t\"Washtenaw County, MI\"\t26161\n\"Oakland County, MI\"\t26125\t\"Wayne County, MI\"\t26163\n\"Oceana County, MI\"\t26127\t\"Lake County, MI\"\t26085\n\"Oceana County, MI\"\t26127\t\"Mason County, MI\"\t26105\n\"Oceana County, MI\"\t26127\t\"Muskegon County, MI\"\t26121\n\"Oceana County, MI\"\t26127\t\"Newaygo County, MI\"\t26123\n\"Oceana County, MI\"\t26127\t\"Oceana County, MI\"\t26127\n\"Oceana County, MI\"\t26127\t\"Ozaukee County, WI\"\t55089\n\"Oceana County, MI\"\t26127\t\"Sheboygan County, WI\"\t55117\n\"Ogemaw County, MI\"\t26129\t\"Alcona County, MI\"\t26001\n\"Ogemaw County, MI\"\t26129\t\"Arenac County, MI\"\t26011\n\"Ogemaw County, MI\"\t26129\t\"Crawford County, MI\"\t26039\n\"Ogemaw County, MI\"\t26129\t\"Gladwin County, MI\"\t26051\n\"Ogemaw County, MI\"\t26129\t\"Iosco County, MI\"\t26069\n\"Ogemaw County, MI\"\t26129\t\"Ogemaw County, MI\"\t26129\n\"Ogemaw County, MI\"\t26129\t\"Oscoda County, MI\"\t26135\n\"Ogemaw County, MI\"\t26129\t\"Roscommon County, MI\"\t26143\n\"Ontonagon County, MI\"\t26131\t\"Gogebic County, MI\"\t26053\n\"Ontonagon County, MI\"\t26131\t\"Houghton County, MI\"\t26061\n\"Ontonagon County, MI\"\t26131\t\"Iron County, MI\"\t26071\n\"Ontonagon County, MI\"\t26131\t\"Keweenaw County, MI\"\t26083\n\"Ontonagon County, MI\"\t26131\t\"Ontonagon County, MI\"\t26131\n\"Ontonagon County, MI\"\t26131\t\"Cook County, MN\"\t27031\n\"Ontonagon County, MI\"\t26131\t\"Ashland County, WI\"\t55003\n\"Osceola County, MI\"\t26133\t\"Clare County, MI\"\t26035\n\"Osceola County, MI\"\t26133\t\"Isabella County, MI\"\t26073\n\"Osceola County, MI\"\t26133\t\"Lake County, MI\"\t26085\n\"Osceola County, MI\"\t26133\t\"Mecosta County, MI\"\t26107\n\"Osceola County, MI\"\t26133\t\"Missaukee County, MI\"\t26113\n\"Osceola County, MI\"\t26133\t\"Newaygo County, MI\"\t26123\n\"Osceola County, MI\"\t26133\t\"Osceola County, MI\"\t26133\n\"Osceola County, MI\"\t26133\t\"Wexford County, MI\"\t26165\n\"Oscoda County, MI\"\t26135\t\"Alcona County, MI\"\t26001\n\"Oscoda County, MI\"\t26135\t\"Alpena County, MI\"\t26007\n\"Oscoda County, MI\"\t26135\t\"Crawford County, MI\"\t26039\n\"Oscoda County, MI\"\t26135\t\"Iosco County, MI\"\t26069\n\"Oscoda County, MI\"\t26135\t\"Montmorency County, MI\"\t26119\n\"Oscoda County, MI\"\t26135\t\"Ogemaw County, MI\"\t26129\n\"Oscoda County, MI\"\t26135\t\"Oscoda County, MI\"\t26135\n\"Oscoda County, MI\"\t26135\t\"Otsego County, MI\"\t26137\n\"Oscoda County, MI\"\t26135\t\"Roscommon County, MI\"\t26143\n\"Otsego County, MI\"\t26137\t\"Antrim County, MI\"\t26009\n\"Otsego County, MI\"\t26137\t\"Charlevoix County, MI\"\t26029\n\"Otsego County, MI\"\t26137\t\"Cheboygan County, MI\"\t26031\n\"Otsego County, MI\"\t26137\t\"Crawford County, MI\"\t26039\n\"Otsego County, MI\"\t26137\t\"Kalkaska County, MI\"\t26079\n\"Otsego County, MI\"\t26137\t\"Montmorency County, MI\"\t26119\n\"Otsego County, MI\"\t26137\t\"Oscoda County, MI\"\t26135\n\"Otsego County, MI\"\t26137\t\"Otsego County, MI\"\t26137\n\"Ottawa County, MI\"\t26139\t\"Allegan County, MI\"\t26005\n\"Ottawa County, MI\"\t26139\t\"Kent County, MI\"\t26081\n\"Ottawa County, MI\"\t26139\t\"Muskegon County, MI\"\t26121\n\"Ottawa County, MI\"\t26139\t\"Ottawa County, MI\"\t26139\n\"Ottawa County, MI\"\t26139\t\"Milwaukee County, WI\"\t55079\n\"Ottawa County, MI\"\t26139\t\"Racine County, WI\"\t55101\n\"Presque Isle County, MI\"\t26141\t\"Alpena County, MI\"\t26007\n\"Presque Isle County, MI\"\t26141\t\"Cheboygan County, MI\"\t26031\n\"Presque Isle County, MI\"\t26141\t\"Chippewa County, MI\"\t26033\n\"Presque Isle County, MI\"\t26141\t\"Mackinac County, MI\"\t26097\n\"Presque Isle County, MI\"\t26141\t\"Montmorency County, MI\"\t26119\n\"Presque Isle County, MI\"\t26141\t\"Presque Isle County, MI\"\t26141\n\"Roscommon County, MI\"\t26143\t\"Clare County, MI\"\t26035\n\"Roscommon County, MI\"\t26143\t\"Crawford County, MI\"\t26039\n\"Roscommon County, MI\"\t26143\t\"Gladwin County, MI\"\t26051\n\"Roscommon County, MI\"\t26143\t\"Kalkaska County, MI\"\t26079\n\"Roscommon County, MI\"\t26143\t\"Missaukee County, MI\"\t26113\n\"Roscommon County, MI\"\t26143\t\"Ogemaw County, MI\"\t26129\n\"Roscommon County, MI\"\t26143\t\"Oscoda County, MI\"\t26135\n\"Roscommon County, MI\"\t26143\t\"Roscommon County, MI\"\t26143\n\"Saginaw County, MI\"\t26145\t\"Bay County, MI\"\t26017\n\"Saginaw County, MI\"\t26145\t\"Genesee County, MI\"\t26049\n\"Saginaw County, MI\"\t26145\t\"Gratiot County, MI\"\t26057\n\"Saginaw County, MI\"\t26145\t\"Midland County, MI\"\t26111\n\"Saginaw County, MI\"\t26145\t\"Saginaw County, MI\"\t26145\n\"Saginaw County, MI\"\t26145\t\"Shiawassee County, MI\"\t26155\n\"Saginaw County, MI\"\t26145\t\"Tuscola County, MI\"\t26157\n\"St. Clair County, MI\"\t26147\t\"Lapeer County, MI\"\t26087\n\"St. Clair County, MI\"\t26147\t\"Macomb County, MI\"\t26099\n\"St. Clair County, MI\"\t26147\t\"St. Clair County, MI\"\t26147\n\"St. Clair County, MI\"\t26147\t\"Sanilac County, MI\"\t26151\n\"St. Joseph County, MI\"\t26149\t\"Elkhart County, IN\"\t18039\n\"St. Joseph County, MI\"\t26149\t\"LaGrange County, IN\"\t18087\n\"St. Joseph County, MI\"\t26149\t\"Branch County, MI\"\t26023\n\"St. Joseph County, MI\"\t26149\t\"Calhoun County, MI\"\t26025\n\"St. Joseph County, MI\"\t26149\t\"Cass County, MI\"\t26027\n\"St. Joseph County, MI\"\t26149\t\"Kalamazoo County, MI\"\t26077\n\"St. Joseph County, MI\"\t26149\t\"St. Joseph County, MI\"\t26149\n\"St. Joseph County, MI\"\t26149\t\"Van Buren County, MI\"\t26159\n\"Sanilac County, MI\"\t26151\t\"Huron County, MI\"\t26063\n\"Sanilac County, MI\"\t26151\t\"Lapeer County, MI\"\t26087\n\"Sanilac County, MI\"\t26151\t\"St. Clair County, MI\"\t26147\n\"Sanilac County, MI\"\t26151\t\"Sanilac County, MI\"\t26151\n\"Sanilac County, MI\"\t26151\t\"Tuscola County, MI\"\t
